vi "RSZVB Get Power Meter Frequency Conversion.vi"(8 "error in (no error)":errorcluster {"code" format="%.0x"}, 9 "Power Meter Number (1)":i32=1, 10 "Channel (1)":i32=1, 11 "VISA session":refnum<visa-resource-name>) -> (0 "error out":errorcluster {"code" format="%.0x"}, 2 "Numerator":i32, 3 "dup VISA session":refnum<visa-resource-name>, 4 "Sweep Type":i32, 5 "Offset":dbl format="%^.3e", 7 "Denominator":i32)   [LabVIEW 2011]
doc: "This VI returns the receiver frequency for frequency-converting measurements. The receiver frequency is either a range (for frequency sweeps) or a CW frequency (for power, time and CW Mode sweeps). The receiver frequency is valid for all ports. \n\nNote(s):\n\n(1) This VI is available only on R&S ZVA instrument.\n\nRemote-control command(s):\n[SENSe<Ch>:]FREQuency:CONVersion:ARBitrary:PMETer<Mtr>?"
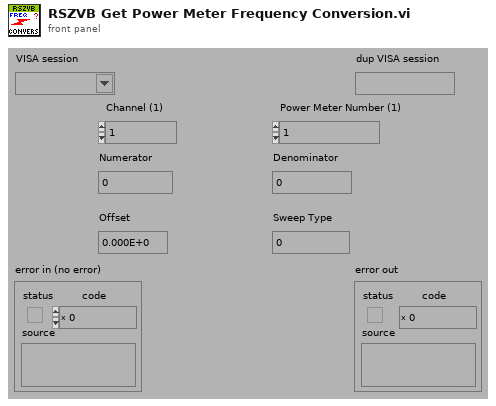
[diagram p1: front panel]
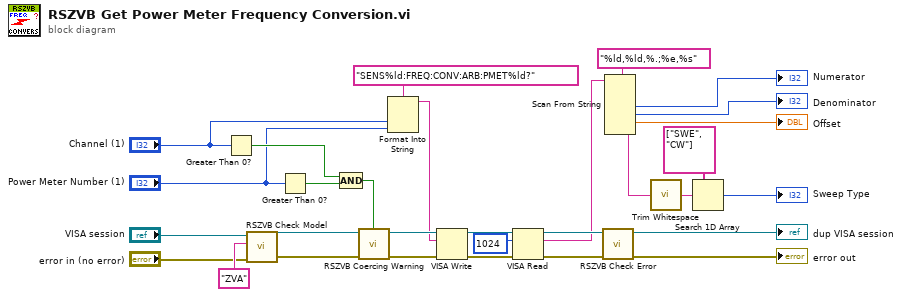
[diagram p0: block diagram]
diagram:
  n1 = Greater Than 0?(x="Channel (1)") -> (x > 0?=w6:bool)
  n2 = call "RSZVB Check Model.vi"("error in (no error)"="error in (no error)", "Model"="ZVA" ("Options"), "VISA session"="VISA session") -> ("error out"=w17:errorcluster, "dup VISA session"=w16:refnum<visa-resource-name>)  [unwired: 7 in]
  n3 = Greater Than 0?(x="Power Meter Number (1)") -> (x > 0?=w4:bool)
  n4 = Compound Arithmetic op=AND(w6, w4) -> (w30:bool)
  n5 = call "RSZVB Coercing Warning.vi"("In Range?"=w30, "error in (no error)"=w17, "VISA session"=w16) -> ("error out"=w29:errorcluster, "dup VISA session"=w28:refnum<visa-resource-name>)  [unwired: 7 in]
  n6 = Format Into String(format string="SENS%ld:FREQ:CONV:ARB:PMET%ld?", "Channel (1)", "Power Meter Number (1)") -> (resulting string=w5:string)  [unwired: 2 in, 1 out]
  n7 = VISA Write(VISA resource name=w28, write buffer=w5, error in (no error)=w29) -> (VISA resource name out=w22:refnum<visa-resource-name>, error out=w23:errorcluster)  [unwired: 1 out]
  n8 = VISA Read(VISA resource name=w22, byte count=u32 1024 ("byte count (0)"), error in (no error)=w23) -> (VISA resource name out=w26:refnum<visa-resource-name>, read buffer=w18:string, error out=w25:errorcluster)  [unwired: 1 out]
  n9 = call "RSZVB Check Error.vi"("error in (no error)"=w25, "VISA session"=w26) -> ("error out"=→"error out":errorcluster, "dup VISA session"=→"dup VISA session":refnum<visa-resource-name>)  [unwired: 8 in]
  n10 = Scan From String(format string="%ld,%ld,%.;%e,%s", input string=w18) -> (output 1=→"Numerator":i32, output 2=→"Denominator":i32, output 3=→"Offset":dbl, output 4=w19:string)  [unwired: 6 in, 3 out]
  n11 = call <vilib>:"Trim Whitespace.vi"("string"=w19) -> ("trimmed string"=w20:string)  [unwired: 1 in]
  n12 = Search 1D Array(1D array=string[] ["SWE", "CW"] ("array 2"), element=w20) -> (index of element=→"Sweep Type":i32)  [unwired: 1 in]
